vi "ShowToolTips.vi"(5 "error in (no error)":errorcluster) -> (19 "error out":errorcluster)   [LabVIEW 2012, in "UmlEditor.lvclass"]
uses:
  <resource>/Framework/Providers/Open_GDS/UML/UmlEditor_class/UmlEditor.lvclass
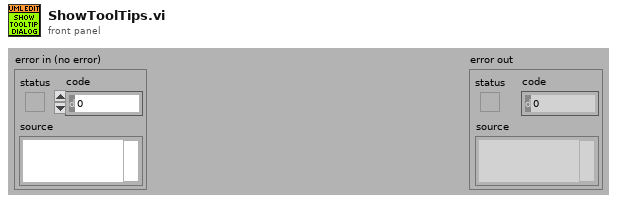
[diagram p1: front panel]
types:
  T1 = enum32{"Bad", "Idle", "Run top level", "Running"}
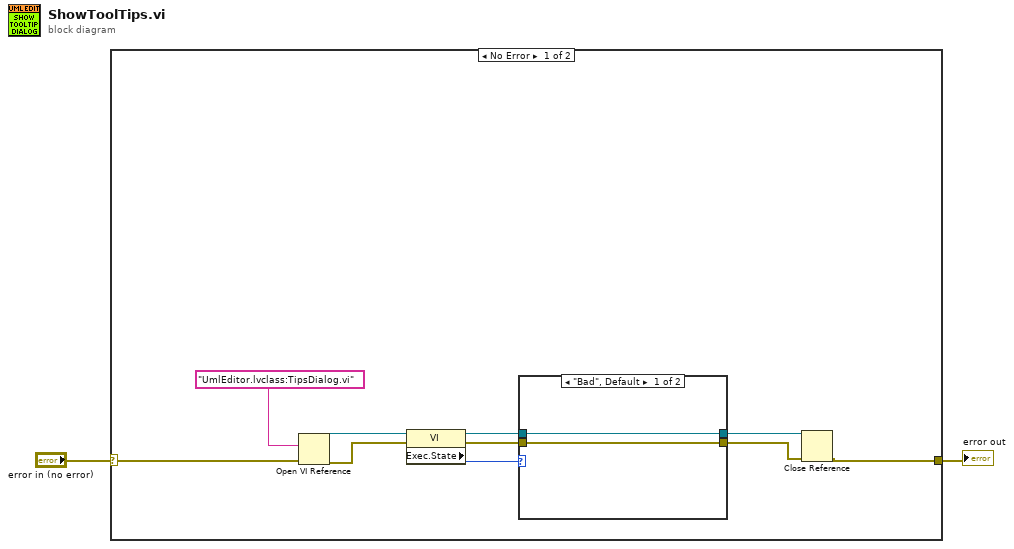
[diagram p0: block diagram]
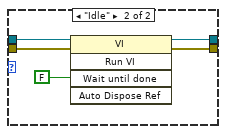
[diagram p2: hidden frame]
diagram:
  n1 = case shown="No Error" "error in (no error)" {
    selector: "error in (no error)" -> [w12 w20]
    tunnel: [w9 w20] -> w1
    frame No Error {
      n2 = Open VI Reference(vi path="UmlEditor.lvclass:TipsDialog.vi", error in (no error)=w12) -> (vi reference=w7:refnum<vi>, error out=w6:errorcluster)  [unwired: 4 out]
      n3 = property class="VI"(reference=w7, error in=w6) -> (reference out=w5:refnum<vi>, error out=w4:errorcluster, "Exec.State"=w3:T1)
      n4 = case shown="\"Bad\", Default" w3 {
        tunnel: [w14 w18] -> w11
        tunnel: [w13 w17] -> w10
        tunnel: w5 -> [w14 w16]
        tunnel: w4 -> [w13 w15]
        frame "Bad", Default {
        }
        frame "Idle" {
          n5 = invoke class="VI" method="Run VI"(reference=w16, error in=w15, "Wait until done"=FALSE ("Wait Until Done")) -> (reference out=w18:refnum<vi>, error out=w17:errorcluster)  [unwired: 2 in, 3 out]
        }
      }
      n6 = Close Reference(reference=w11, error in (no error)=w10) -> (error out=w9:errorcluster)
    }
    frame Error {
    }
  }
  "error out" <- w1
